vi "SVX Create Waterfall Cursor.vi"   [LabVIEW 2016]
doc: "This VI creates a line that you can plot on a waterfall graph. Use the waterfall graph property node <B>lines</B> to draw the line on the graph."
uses:
  <vilib>/addons/_XControls/Utility/subVIs/svx_Waterfall Frequency Cursor.vi
  <vilib>/addons/_XControls/Waterfall Graph/SVX Waterfall Graph.xctl
types:
  T1 = typedef "svc_Cluster of Array of Cluster of XYZ.ctl" = cluster{"line":cluster{"X":dbl, "Y":dbl, "Z":dbl}[]}
  T2 = cluster{"z0":dbl, "dz":dbl, "plots":cluster{"x0":dbl, "dx":dbl, "Y":dbl[]}[]}
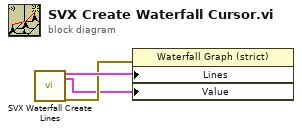
[diagram p0: block diagram]
diagram:
  n1 = call-poly <vilib>:"SVX Waterfall Create Lines.vi"() -> ("appended cursors"=w3:T1[], "duplicate waterfall data"=w1:T2, "error out"=w2:errorcluster)  [unwired: 14 in, 3 out]
  n2 = property on="Property Node" class="Waterfall Graph (strict)"(error in=w2, "Lines"=w3, "Value"=w1) -> ()  [unwired: 1 in, 2 out]
